vi "Delete Message Template Files.vi"(8 "error in (no error)":errorcluster, 11 "Library":refnum<vi>) -> (0 "error out":errorcluster, 3 "Library":refnum<vi>)   [LabVIEW 2019, in "gRPC Template Creation Utility.lvlib"]
uses:
  gRPC Template Creation Utility.lvlib
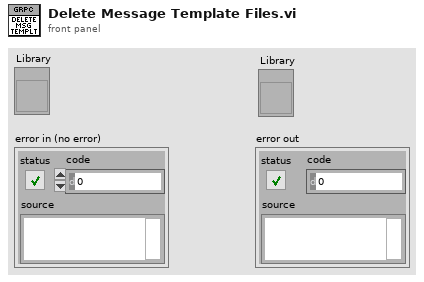
[diagram p1: front panel]
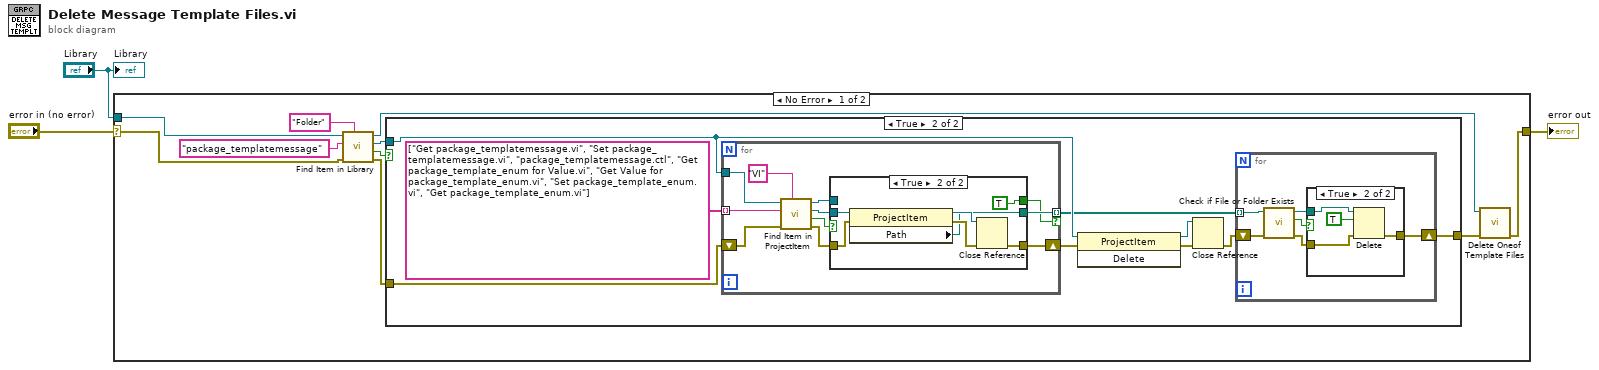
[diagram p0: block diagram]
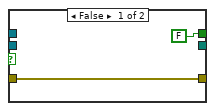
[diagram p4: hidden frame]
diagram:
  n1 = case shown="No Error" "error in (no error)" {
    selector: "error in (no error)" -> [w7 w55]
    tunnel: "Library" -> [w11 _]
    tunnel: [w4 w55] -> w1
    frame No Error {
      n2 = call "Find Item in Library.vi"("Item Type"="Folder", "error in (no error)"=w7, "Item Name"="package_templatemessage", "Library item in"=w11) -> ("error out"=w9:errorcluster, "Found?"=w8:bool, "Project Item (Library Item)"=w10:refnum<vi>, "Library item out"=w5:refnum<vi>)  [unwired: 4 in]
      n3 = case shown="True" w8 {
        tunnel: w10 -> [_ w19]
        tunnel: w9 -> [w14 w23]
        tunnel: [w14 w15] -> w6
        frame False {
        }
        frame True {
          n4 = for {
            tunnel: w19 -> [w45]
            shift-right: [w38] -> w20
            shift-left: w23 -> [w40]
            tunnel: string[] ["Get package_templatemessage.vi", "Set package_templatemessage.vi", "package_templatemessage.ctl", "Get package_template_enum for Value.vi", "Get Value for package_template_enum.vi", "Set package_template_enum.vi", "Get package_template_enum.vi"] -> [w37] mode=indexing
            tunnel: [w36] -> w16 mode=indexing if=w35
            n5 = call "Find Item in ProjectItem.vi"("Item Type"="VI", "error in (no error)"=w40, "Name"=w37, "ProjectItem in"=w45) -> ("error out"=w39:errorcluster, "Found ?"=w43:bool, "Item Refnum out"=w41:refnum<vi>, "ProjectItem out"=w42:refnum<vi>)  [unwired: 4 in]
            n6 = case shown="True" w43 {
              tunnel: w39 -> [w47 w54]
              tunnel: w41 -> [_ w53]
              tunnel: w42 -> [_ _]
              tunnel: [w47 w48] -> w38
              tunnel: [_ w50] -> w36
              tunnel: [FALSE TRUE] -> w35
              frame False {
              }
              frame True {
                n7 = property class="ProjectItem"(reference=w53, error in=w54) -> (reference out=w52:refnum<vi>, error out=w51:errorcluster, "Path"=w50:path)
                n8 = Close Reference(reference=w52, error in (no error)=w51) -> (error out=w48:errorcluster)
              }
            }
          }
          n9 = invoke class="ProjectItem" method="Delete"(reference=w19, error in=w20) -> (reference out=w22:refnum<vi>, error out=w21:errorcluster)  [unwired: 1 in, 1 out]
          n10 = Close Reference(reference=w22, error in (no error)=w21) -> (error out=w17:errorcluster)
          n11 = for {
            shift-right: [w25] -> w15
            shift-left: w17 -> [w26]
            tunnel: w16 -> [w24] mode=indexing
            n12 = call <vilib>:"Check if File or Folder Exists.vi"("error in (no error)"=w26, "path"=w24) -> ("error out"=w29:errorcluster, "file or folder exists?"=w27:bool, "dup path"=w28:path)  [unwired: 7 in]
            n13 = case shown="True" w27 {
              tunnel: w28 -> [_ w34]
              tunnel: w29 -> [w30 w33]
              tunnel: [w30 w32] -> w25
              frame False {
              }
              frame True {
                n14 = Delete(path (use dialog)=w34, entire hierarchy (F)=TRUE, error in=w33) -> (error out=w32:errorcluster)  [unwired: 2 in, 2 out]
              }
            }
          }
        }
      }
      n15 = call "Delete Oneof Template Files.vi"("error in (no error)"=w6, "Library in"=w5) -> ("error out"=w4:errorcluster)  [unwired: 8 in, 1 out]
    }
    frame Error {
    }
  }
  "error out" <- w1
  "Library" <- "Library"
